vi "exercicios12_dui.vi"() -> ()   [LabVIEW 2018]
panel:
  in  "?":bool
  out "?":dbl
  in  "Mensagem":string
  in  "Número":string
  in  "Nome":string
  in  "?":bool
  out "Waveform Chart":dbl[](graph)
  in  "?":bool
  # "Exercício 1"
  # "Exercício 2"
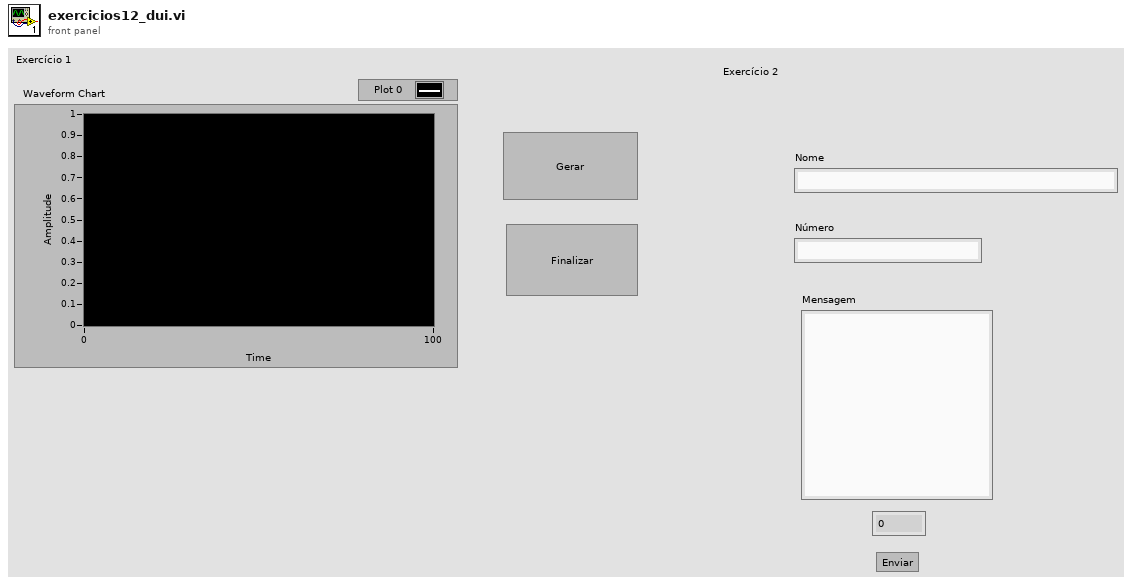
[diagram p1: front panel]
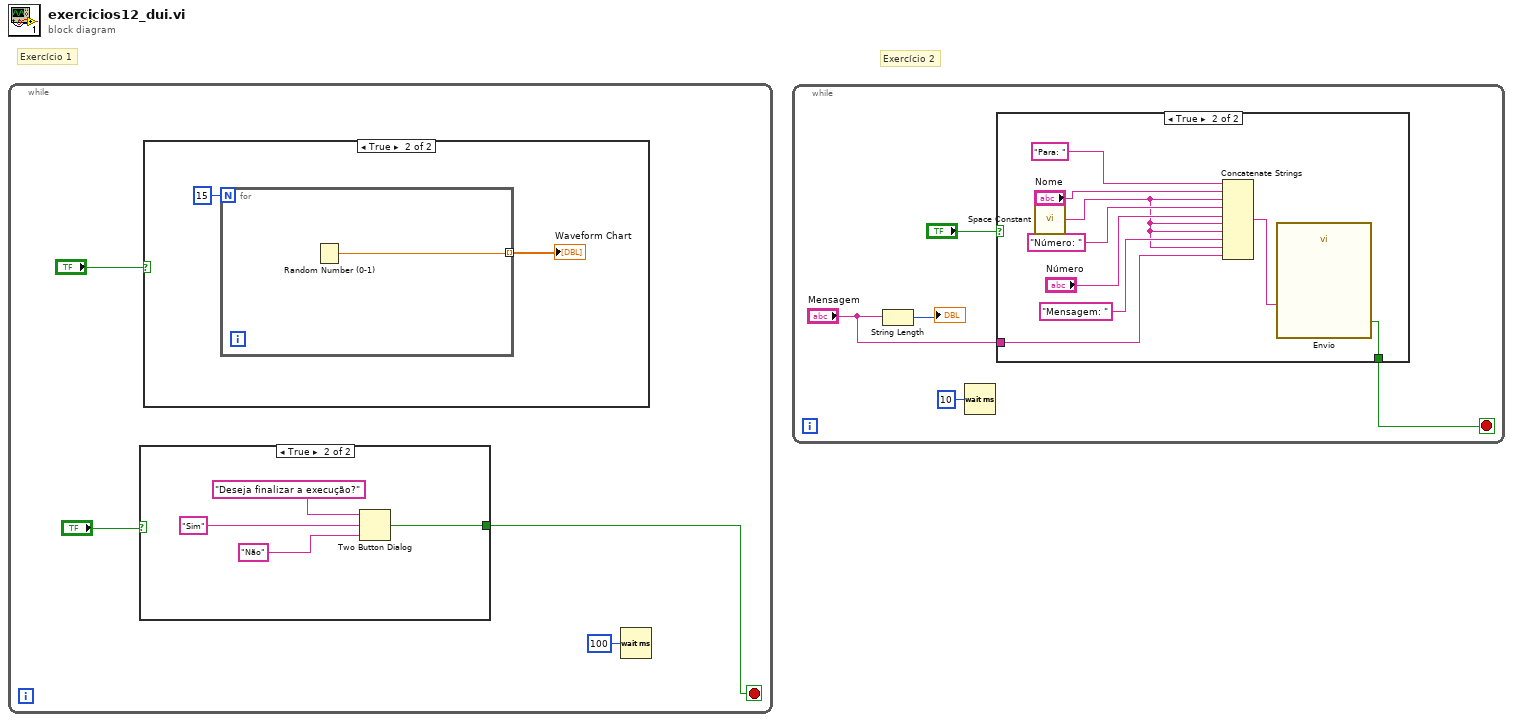
[diagram p0: block diagram]
diagram:
  # "Exercício 2"
  # "Exercício 1"
  n1 = while {
    stop <- w2 stop-if-true
    n2 = case shown="True" "?" {
      tunnel: [_ w5] -> w2
      frame False {
      }
      frame True {
        n3 = Two Button Dialog(message="Deseja finalizar a execução?", 1:"Não" ("F button name (\"Cancel\")"), 2:"Sim" ("T button name (\"OK\")")) -> (T button?=w5:bool)
      }
    }
    n4 = case shown="True" "?" {
      frame False {
      }
      frame True {
        n5 = for {
          N: 15 -> [_]
          tunnel: [w11] -> w9 mode=indexing
          n6 = Random Number (0-1)() -> (number: 0 to 1=w11:dbl)
        }
        "Waveform Chart" <- w9
      }
    }
    n7 = Wait (ms)(milliseconds to wait=u32 100) -> ()  [unwired: 1 out]
  }
  n8 = while {
    stop <- w13 stop-if-true
    n9 = String Length(string="Mensagem") -> (length=→"?":i32)
    n10 = Wait (ms)(milliseconds to wait=u32 10) -> ()  [unwired: 1 out]
    n11 = case shown="True" "?" {
      tunnel: "Mensagem" -> [_ w21]
      tunnel: [_ w19] -> w13
      frame False {
      }
      frame True {
        n12 = call <vilib>:"Space Constant.vi"() -> ("String"=w17:string)
        n13 = Concatenate Strings("Para: " ("string"), "Nome", w17, "Número: " ("string"), "Número", w17, w17, "Mensagem: " ("string"), w17, w21) -> (w20:string)
        n14 = call "Envio"("Message"=w20) -> ("OK"=w19:bool)  [unwired: 9 in, 1 out]
      }
    }
  }
